vi "Read Transport.vi"(11 "Base Spawn in":refnum<class "Base Spawn.lvclass">) -> (2 "Transport":refnum<class "Transport.lvclass">)   [LabVIEW 2025, in "jettl.lvlib" / "Spawn.lvlib" / "Base Spawn.lvclass"]
uses:
  Base Spawn.lvclass
  Base Spawn.lvclass/Base Spawn.ctl
  Transport/Transport/Transport.lvclass
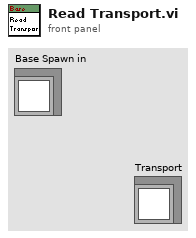
[diagram p1: front panel]
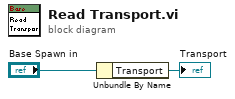
[diagram p0: block diagram]
diagram:
  n1 = Unbundle By Name("Base Spawn in") -> ("Transport"=→"Transport":refnum<class "Transport.lvclass">)
